vi "alignVerticalCenters.vi"(6 "useControlBodyOnly":bool, 8 "error in (no error)":errorcluster, 11 "refs":refnum<vi>[](array[refnum])) -> (0 "error out":errorcluster, 3 "refs(dup)":refnum<vi>[](array[refnum]))   [LabVIEW 2023]
doc: "Aligns all controls to a common vertical center by applying the same Y-center coordinate to each control."
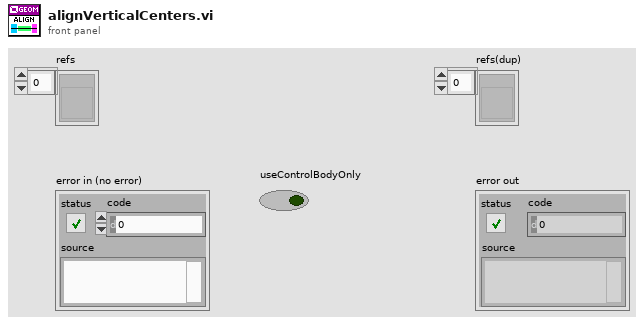
[diagram p1: front panel]
types:
  T1 = cluster{"left":i32, "top":i32, "right":i32, "bottom":i32}
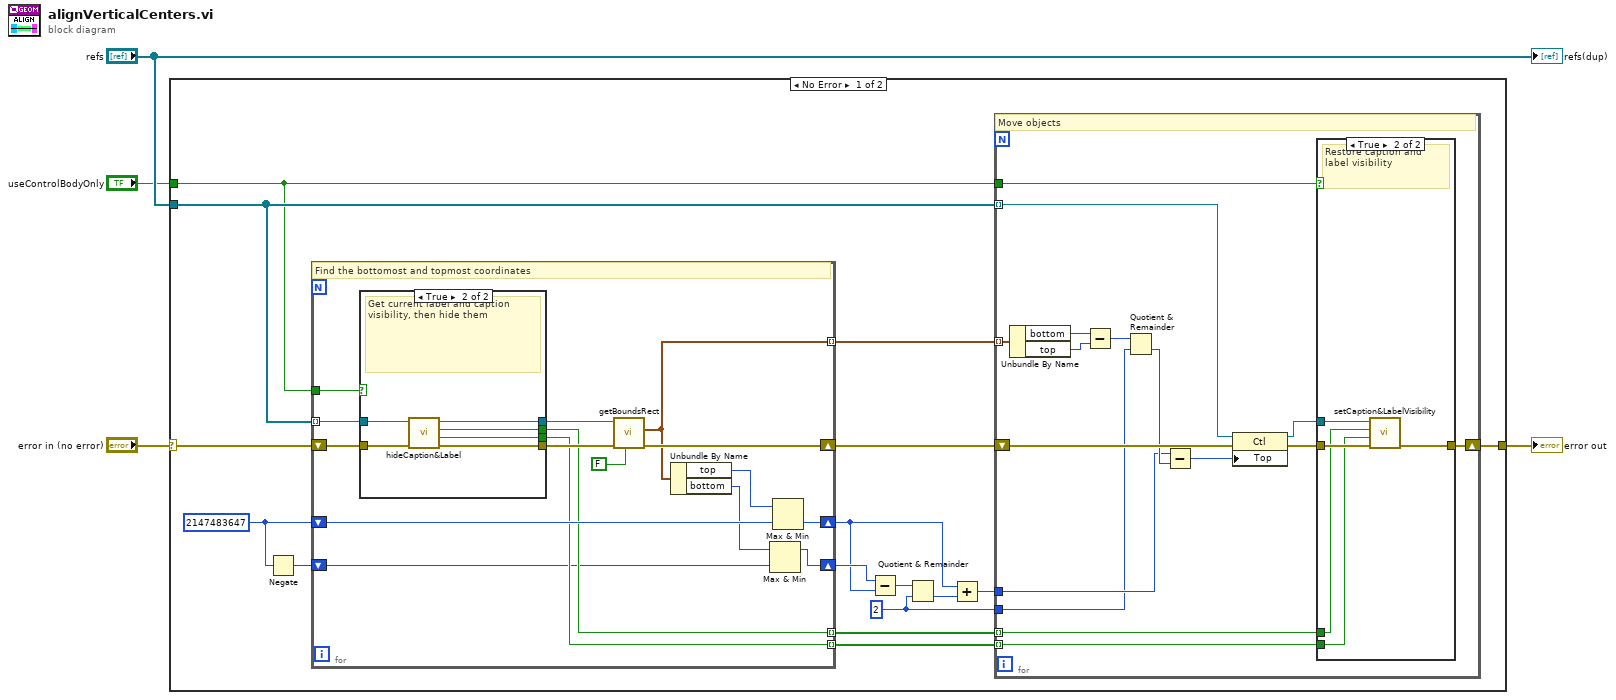
[diagram p0: block diagram]
diagram:
  n1 = case shown="No Error" "error in (no error)" {
    selector: "error in (no error)" -> [w20 w67]
    tunnel: [w19 w67] -> w1
    tunnel: "refs" -> [w6 _]
    tunnel: "useControlBodyOnly" -> [w5 _]
    frame No Error {
      w7 = 2 ("y")
      w14 = 2147483647
      n2 = Negate(x=w14) -> (-x=w13:i32)
      n3 = for {
        tunnel: w6 -> [w54] mode=indexing
        shift-right: [w58] -> w18
        shift-left: w20 -> [w53]
        shift-right: [w45] -> w9
        shift-left: w14 -> [w57]
        tunnel: [w56] -> w17 mode=indexing
        tunnel: w5 -> [w51]
        tunnel: [w50] -> w16 mode=indexing
        tunnel: [w49] -> w15 mode=indexing
        shift-right: [w43] -> w12
        shift-left: w13 -> [w47]
        # "Find the bottomost and topmost coordinates"
        n4 = case shown="True" w51 {
          tunnel: [w60 w64] -> w55
          tunnel: w54 -> [w60 w65]
          tunnel: w53 -> [w59 w66]
          tunnel: [w59 w63] -> w52
          tunnel: [_ w62] -> w50
          tunnel: [_ w61] -> w49
          frame False {
            # "Do nothing"
          }
          frame True {
            # "Get current label and caption visibility, then hide them"
            n5 = call "hideCaption&Label.vi"("error in (no error)"=w66, "Control in"=w65) -> ("error out"=w63:errorcluster, "Label.Visible"=w61:bool, "Caption.Visible"=w62:bool, "Control out"=w64:refnum<vi>)  [unwired: 6 in]
          }
        }
        n6 = call "getBoundsRect.vi"("useControlBodyOnly"=FALSE ("ignoreCaption&Labels"), "error in (no error)"=w52, "ref"=w55) -> ("error out"=w58:errorcluster, "rect"=w56:T1)  [unwired: 6 in, 1 out]
        n7 = Unbundle By Name(w56) -> ("top"=w46:i32, "bottom"=w44:i32)
        n8 = Max & Min(x=w44, y=w47) -> (max(x,y)=w43:i32)  [unwired: 1 out]
        n9 = Max & Min(x=w46, y=w57) -> (min(x,y)=w45:i32)  [unwired: 1 out]
      }
      n10 = Subtract(x=w12, y=w9) -> (x-y=w11:i32)
      n11 = Quotient & Remainder(x=w11, y=w7) -> (floor(x/y)=w10:i32)  [unwired: 1 out]
      n12 = Add(x=w9, y=w10) -> (x+y=w8:i32)
      n13 = for {
        tunnel: w6 -> [w36] mode=indexing
        shift-right: [w30] -> w19
        shift-left: w18 -> [w31]
        tunnel: w17 -> [w35] mode=indexing
        tunnel: w5 -> [w28]
        tunnel: w16 -> [w26] mode=indexing
        tunnel: w15 -> [w25] mode=indexing
        tunnel: w8 -> [w22]
        tunnel: w7 -> [w21]
        # "Move objects"
        n14 = Unbundle By Name(w35) -> ("bottom"=w34:i32, "top"=w33:i32)
        n15 = Subtract(x=w34, y=w33) -> (x-y=w23:i32)
        n16 = Quotient & Remainder(x=w23, y=w21) -> (floor(x/y)=w24:i32)  [unwired: 1 out]
        n17 = Subtract(x=w22, y=w24) -> (x-y=w32:i32)
        n18 = property class="Ctl"(reference=w36, error in=w31, "Top"=w32) -> (reference out=w27:refnum<vi>, error out=w29:errorcluster)
        n19 = case shown="True" w28 {
          tunnel: w27 -> [_ w40]
          tunnel: w29 -> [w37 w42]
          tunnel: [w37 w41] -> w30
          tunnel: w26 -> [_ w39]
          tunnel: w25 -> [_ w38]
          frame False {
            # "Do nothing"
          }
          frame True {
            # "Restore caption and label visibility"
            n20 = call "setCaption&LabelVisibility.vi"("error in (no error)"=w42, "Label.Visible"=w38, "Caption.Visible"=w39, "Control in"=w40) -> ("error out"=w41:errorcluster)  [unwired: 6 in, 1 out]
          }
        }
      }
    }
    frame Error {
    }
  }
  "error out" <- w1
  "refs(dup)" <- "refs"
